vi "Write Error to File.vi"(8 "Error In":errorcluster, 10 "Error code":i32, 11 "string":string) -> (0 "Error Out":errorcluster)   [LabVIEW 2019]
panel:
  out "Error String":string
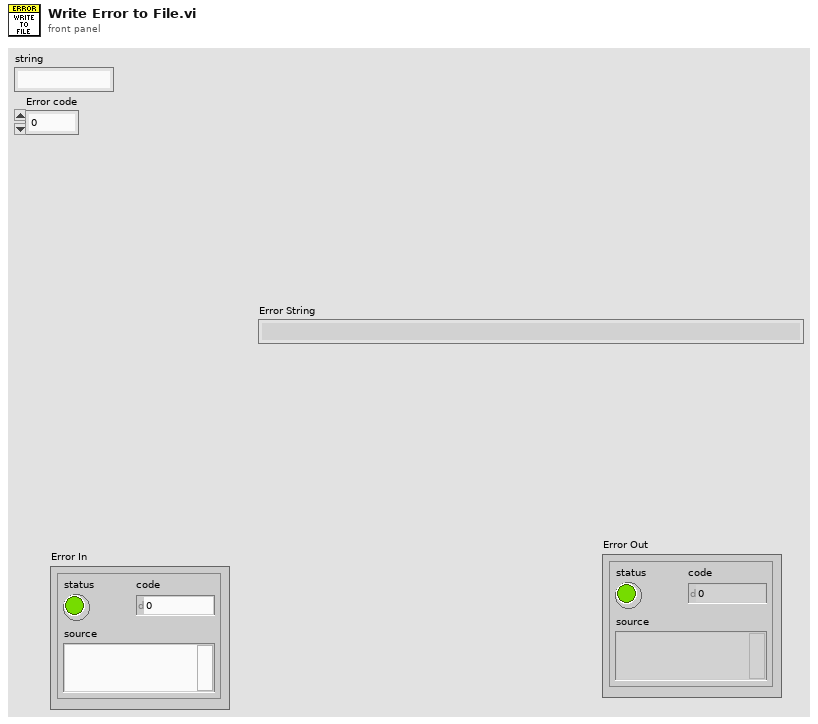
[diagram p1: front panel]
types:
  T1 = enum16{"open", "replace", "create", "open or create", "replace or create", "replace or create with confirmation"}
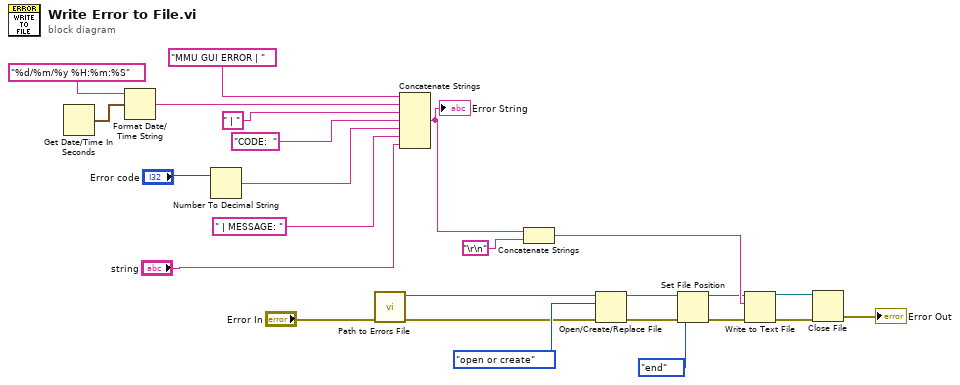
[diagram p0: block diagram]
diagram:
  n1 = Get Date/Time In Seconds() -> (seconds since 1Jan1904=w25:timestamp)
  n2 = Format Date/Time String(time format string (%c)="%d/%m/%y %H:%m:%S", seconds (now)=w25) -> (date/time string=w22:string)  [unwired: 1 in]
  n3 = Number To Decimal String(number="Error code") -> (decimal integer string=w19:string)  [unwired: 1 in]
  n4 = call "Path to Errors File.vi"("Error In"="Error In") -> ("Error Out"=w3:errorcluster, "Path to Errors File"=w4:path)  [unwired: 9 in]
  n5 = Concatenate Strings("MMU GUI ERROR | " ("string"), w22, " | " ("string"), "CODE:  " ("string"), w19, " | MESSAGE: " ("string"), "string") -> (w13:string)
  "Error String" <- w13
  n6 = Concatenate Strings(w13, "\r\n") -> (w12:string)
  n7 = Open/Create/Replace File(file path (use dialog)=w4, error in=w3, operation (0:open)=T1."open or create") -> (refnum out=w7:refnum<file>, error out=w8:errorcluster)  [unwired: 3 in, 1 out]
  n8 = Set File Position(refnum=w7, from (0:start)=enum16{"start", "end", "current"}."end", error in=w8) -> (refnum out=w5:refnum<file>, error out=w6:errorcluster)  [unwired: 1 in]
  n9 = Write to Text File(file (use dialog)=w5, text=w12, error in=w6) -> (refnum out=w11:refnum<file>, error out=w10:errorcluster)  [unwired: 1 in, 1 out]
  n10 = Close File(refnum=w11, error in=w10) -> (error out=→"Error Out":errorcluster)  [unwired: 1 out]
